vi "분석기_누락.vi"() -> ()   [LabVIEW 2014]
uses:
  <vilib>/Utility/file.llb/Read From Spreadsheet File (string).vi
  <vilib>/Utility/file.llb/Read From Spreadsheet File (I64).vi
panel:
  in  "discard_channel":path
  in  "Name":path
  in  "Save_path":path
  in  "Online_Path":path
  in  "Training_Path":path
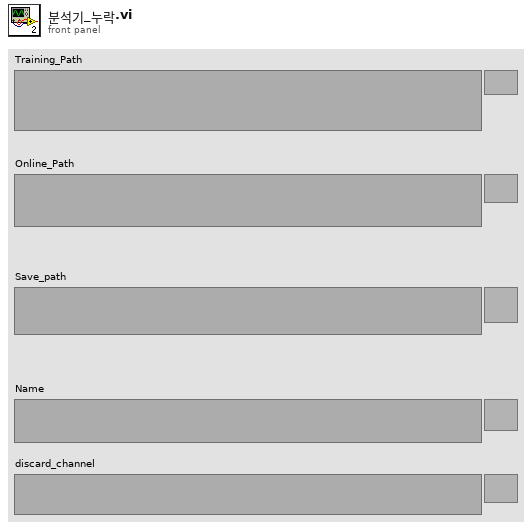
[diagram p1: front panel]
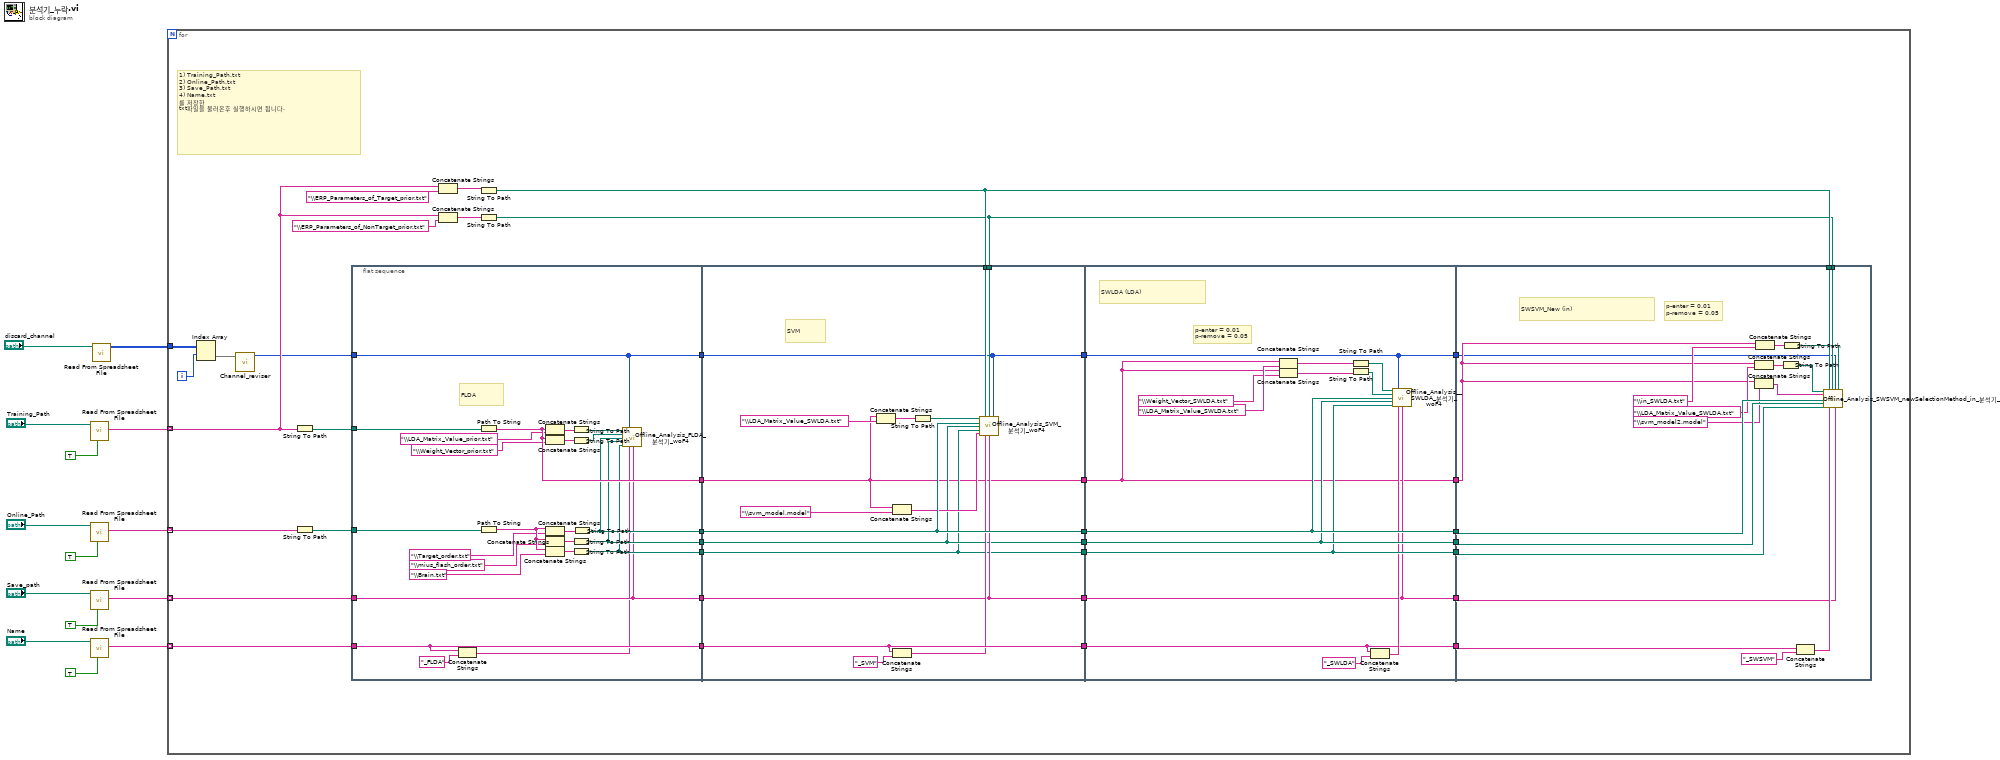
[diagram p0: block diagram]
diagram:
  n1 = call-poly <vilib>:"Read From Spreadsheet File.vi"("transpose (no:F)"=TRUE, "file path (dialog if empty)"="Training_Path") -> ("first row"=w12:string[])  [unwired: 5 in, 4 out]
  n2 = call-poly <vilib>:"Read From Spreadsheet File.vi"("transpose (no:F)"=TRUE, "file path (dialog if empty)"="Online_Path") -> ("first row"=w9:string[])  [unwired: 5 in, 4 out]
  n3 = call-poly <vilib>:"Read From Spreadsheet File.vi"("transpose (no:F)"=TRUE, "file path (dialog if empty)"="Save_path") -> ("first row"=w6:string[])  [unwired: 5 in, 4 out]
  n4 = call-poly <vilib>:"Read From Spreadsheet File.vi"("transpose (no:F)"=TRUE, "file path (dialog if empty)"="Name") -> ("first row"=w3:string[])  [unwired: 5 in, 4 out]
  n5 = call-poly <vilib>:"Read From Spreadsheet File.vi"("file path (dialog if empty)"="discard_channel") -> ("all rows"=w1:i64[][])  [unwired: 6 in, 4 out]
  n6 = for {
    tunnel: w12 -> [w29] mode=indexing
    tunnel: w9 -> [w35] mode=indexing
    tunnel: w6 -> [w33] mode=indexing
    tunnel: w3 -> [w22] mode=indexing
    tunnel: w1 -> [w20]
    i -> [w19]
    # "1) Training_Path.txt\n2) Online_Path.txt\n3) Save_Path.txt\n4) Name.txt\n를 저장한\ntxt파일을 불러온후 실행하시면 됩니다."
    n7 = Index Array(array=w20, index (row)=w19) -> (element=w21:i64[])  [unwired: 1 in]
    n8 = call "Channel_reviser.vi"("CHANNEL_ARRAY"=w21) -> ("CHANNEL_ARRAY_revised"=w18:i64[])  [unwired: 10 in]
    n9 = String To Path(string=w29) -> (path=w36:path)
    n10 = String To Path(string=w35) -> (path=w34:path)
    n11 = flat-sequence {
      tunnel: [w75] -> w51
      tunnel: [w74] -> w50
      tunnel: [w73] -> w49
      tunnel: [w72] -> w48
      tunnel: [w71] -> w47
      tunnel: [w70] -> w30
      tunnel: w33 -> [w70]
      tunnel: w22 -> [w75]
      tunnel: w34 -> [w68]
      tunnel: w36 -> [w69]
      tunnel: w18 -> [w52]
      tunnel: [w52] -> w17
      tunnel: w51 -> [w88]
      tunnel: [w88] -> w46
      tunnel: w50 -> [w78]
      tunnel: [w78] -> w45
      tunnel: w49 -> [w91]
      tunnel: [w91] -> w44
      tunnel: w48 -> [w81]
      tunnel: [w81] -> w43
      tunnel: w47 -> [w80]
      tunnel: [w80] -> w42
      tunnel: [w85] -> w31
      tunnel: w30 -> [w85]
      tunnel: w24 -> [w84]
      tunnel: w23 -> [w83]
      tunnel: w17 -> [w76]
      tunnel: [w76] -> w16
      tunnel: [w101] -> w41
      tunnel: [w95] -> w40
      tunnel: [w106] -> w39
      tunnel: [w105] -> w38
      tunnel: [w104] -> w37
      tunnel: [w100] -> w32
      tunnel: w31 -> [w100]
      tunnel: w42 -> [w104]
      tunnel: w43 -> [w105]
      tunnel: w44 -> [w106]
      tunnel: w45 -> [w95]
      tunnel: w46 -> [w101]
      tunnel: w16 -> [w92]
      tunnel: [w92] -> w15
      tunnel: w32 -> [w117]
      tunnel: w37 -> [w122]
      tunnel: w38 -> [w118]
      tunnel: w39 -> [w123]
      tunnel: w40 -> [w108]
      tunnel: w41 -> [w121]
      tunnel: w23 -> [w120]
      tunnel: w24 -> [w119]
      tunnel: w15 -> [w107]
      frame #0 {
        # "FLDA"
        n12 = Concatenate Strings(w75, "_FLDA" ("string")) -> (w66:string)
        n13 = Path To String(path=w69) -> (string=w74:string)
        n14 = Path To String(path=w68) -> (string=w65:string)
        n15 = Concatenate Strings(w74, "\\LDA_Matrix_Value_prior.txt" ("string")) -> (w56:string)
        n16 = Concatenate Strings(w74, "\\Weight_Vector_prior.txt" ("string")) -> (w55:string)
        n17 = Concatenate Strings(w65, "\\Target_order.txt" ("string")) -> (w61:string)
        n18 = Concatenate Strings(w65, "\\mius_flash_order.txt" ("string")) -> (w60:string)
        n19 = Concatenate Strings(w65, "\\Brain.txt" ("string")) -> (w59:string)
        n20 = String To Path(string=w56) -> (path=w54:path)
        n21 = String To Path(string=w55) -> (path=w53:path)
        n22 = String To Path(string=w60) -> (path=w72:path)
        n23 = String To Path(string=w59) -> (path=w71:path)
        n24 = String To Path(string=w61) -> (path=w73:path)
        n25 = call "Offline_Analysis_FLDA_분석기_woF4.vi"("LDA_matrix"=w54, "DIscard Channel Info"=w52, "Weight"=w53, "Target_order.txt"=w73, "mius_flash_order"=w72, "Brain"=w71, "피험자이름"=w66, "Save_path"=w70) -> ()  [unwired: 8 in]
      }
      frame #1 {
        # "SVM"
        n26 = Concatenate Strings(w78, "\\LDA_Matrix_Value_SWLDA.txt" ("string")) -> (w77:string)
        n27 = Concatenate Strings(w78, "\\svm_model.model" ("string")) -> (w86:string)
        n28 = Concatenate Strings(w88, "_SVM" ("string")) -> (w87:string)
        n29 = String To Path(string=w77) -> (path=w82:path)
        n30 = call "Offline_Analysis_SVM_분석기_woF4.vi"("LDA_matrix"=w82, "Target"=w84, "Nontarget"=w83, "DIscard Channel Info"=w76, "Target_order.txt"=w91, "mius_flash_order"=w81, "Brain"=w80, "svm_model_file"=w86, "피험자이름"=w87, "Save_path"=w85) -> ()  [unwired: 6 in]
      }
      frame #2 {
        # "p-enter = 0.01\np-remove = 0.05"
        # "SWLDA (LDA)"
        n31 = Concatenate Strings(w95, "\\LDA_Matrix_Value_SWLDA.txt") -> (w94:string)
        n32 = Concatenate Strings(w95, "\\Weight_Vector_SWLDA.txt") -> (w93:string)
        n33 = String To Path(string=w94) -> (path=w99:path)
        n34 = String To Path(string=w93) -> (path=w98:path)
        n35 = Concatenate Strings(w101, "_SWLDA" ("string")) -> (w102:string)
        n36 = call "Offline_Analysis__SWLDA_분석기_woF4.vi"("LDA_matrix"=w99, "DIscard Channel Info"=w92, "Weight"=w98, "Target_order.txt"=w106, "mius_flash_order"=w105, "Brain"=w104, "피험자이름"=w102, "Save_path"=w100) -> ()  [unwired: 8 in]
      }
      frame #3 {
        # "p-enter = 0.01\np-remove = 0.05"
        # "SWSVM_New (in)"
        n37 = Concatenate Strings(w108, "\\svm_model2.model") -> (w113:string)
        n38 = Concatenate Strings(w108, "\\LDA_Matrix_Value_SWLDA.txt") -> (w111:string)
        n39 = Concatenate Strings(w108, "\\in_SWLDA.txt") -> (w112:string)
        n40 = String To Path(string=w111) -> (path=w115:path)
        n41 = String To Path(string=w112) -> (path=w110:path)
        n42 = Concatenate Strings(w121, "_SWSVM" ("string")) -> (w125:string)
        n43 = call "Offline_Analysis_SWSVM_newSelectionMethod_in_분석기_woF4.vi"("LDA_matrix"=w115, "svm_model_file"=w113, "Target_order.txt"=w123, "mius_flash_order"=w118, "Brain"=w122, "Target"=w119, "피험자이름"=w125, "Nontarget"=w120, "DIscard Channel Info"=w107, "Save_path"=w117, "in_matrix"=w110) -> ()  [unwired: 9 in]
      }
    }
    n44 = Concatenate Strings(w29, "\\ERP_Parameters_of_Target_prior.txt" ("string")) -> (w26:string)
    n45 = Concatenate Strings(w29, "\\ERP_Parameters_of_NonTarget_prior.txt" ("string")) -> (w25:string)
    n46 = String To Path(string=w26) -> (path=w24:path)
    n47 = String To Path(string=w25) -> (path=w23:path)
  }
